vi "Type Color.vi"(11 "MySquare in":refnum<class "MySquare.lvclass">) -> (2 "Type Color":u32(colorbox)=9868950)   [LabVIEW 2020]
uses:
  MySquare.lvclass
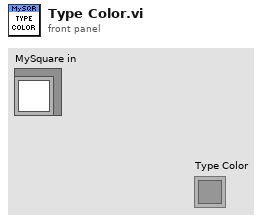
[diagram p1: front panel]
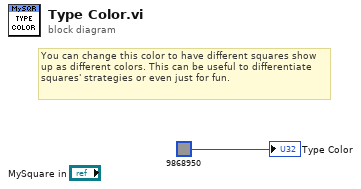
[diagram p0: block diagram]
diagram:
  # "You can change this color to have different squares show up as different colors. This can be useful to differentiate squares' strategies or even just for fun."
  "Type Color" <- u32 9868950 ("Type Color")
